vi "Load_Position.vi"(4 "Relative?":bool, 6 "Error In":errorcluster, 7 "Position":i64, 8 "Node":i32, 9 "Serial In":refnum<visa-resource-name>) -> (0 "Error Out":errorcluster, 3 "Serial Out":refnum<visa-resource-name>)   [LabVIEW 2019]
uses:
  <vilib>/Utility/error.llb/Error Cluster From Error Code.vi
  <vilib>/ErrorRing/Error Ring.xnode
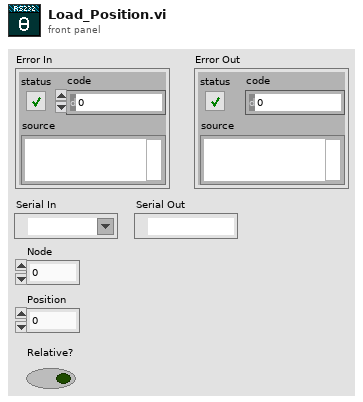
[diagram p1: front panel]
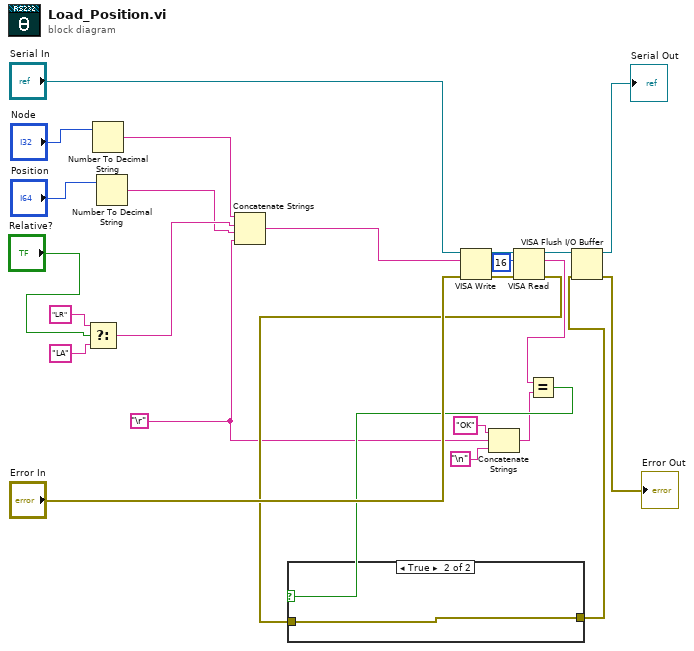
[diagram p0: block diagram]
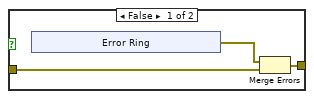
[diagram p2: hidden frame]
diagram:
  w4 = "\r"
  n1 = Select(t="LR", s="Relative?", f="LA") -> (s? t:f=w17:string)
  n2 = Number To Decimal String(number="Node") -> (decimal integer string=w18:string)  [unwired: 1 in]
  n3 = Number To Decimal String(number="Position") -> (decimal integer string=w16:string)  [unwired: 1 in]
  n4 = Concatenate Strings(w18, w17, w16, w4) -> (w15:string)
  n5 = VISA Write(VISA resource name="Serial In", write buffer=w15, error in (no error)="Error In") -> (VISA resource name out=w12:refnum<visa-resource-name>, error out=w11:errorcluster)  [unwired: 1 out]
  n6 = Concatenate Strings("OK" ("y"), w4, "\n") -> (w2:string)
  n7 = VISA Read(VISA resource name=w12, byte count=u32 16, error in (no error)=w11) -> (VISA resource name out=w9:refnum<visa-resource-name>, read buffer=w8:string, error out=w6:errorcluster)  [unwired: 1 out]
  n8 = Equal?(x=w8, y=w2) -> (x = y?=w7:bool)
  n9 = case shown="True" w7 {
    tunnel: w6 -> [w27 w34]
    tunnel: [w28 w34] -> w5
    frame False {
      n10 = xnode "Error Ring"() -> ("error out"=w26:errorcluster)
      n11 = Merge Errors(w26, w27) -> (w28:errorcluster)
    }
    frame True {
    }
  }
  n12 = VISA Flush I/O Buffer(VISA resource name=w9, error in (no error)=w5) -> (VISA resource name out=→"Serial Out":refnum<visa-resource-name>, error out=→"Error Out":errorcluster)  [unwired: 1 in]
